vi "EntêteFichierTlog.vi"(3 "Error in":errorcluster, 4 "TSensPAr":T1[](array[typedef]) {"Compensation" items=["Off", "On"]; "TableConv" max=60 step=1; "Type" items=["Silicon Diode", "GaAlAs Diode", "Platinum 100 (250 Ohms)", "Platinum 100 (500 Ohms)", "Platinum 1000 Ohms", "NTC RTD 75mV 7.5 KOhms", "Thermocouple 25mV", "Thermocouple 50mV", "NTC RTD 75mV 75 Ohms", "NTC RTD 75mV 750 Ohms", "NTC RTD 75mV 7.5 KOhms", "NTC RTD 75mV 75 KOhms", "NTC RTD 75mV Auto"]; "TableTC" max=41 step=1}, 5 "ConfigChoisies":string[](array[string]) caption="Configurations\nChoisies") -> (0 "error out":errorcluster, 1 "Entête":string, 2 "Scan list Out":string[](array[string]))   [LabVIEW 2010]
doc: "Ce Vi créer la ligne d'entête du fichier texte de sauvegarde à partir du nombre de paramètre voulus."
uses:
  <userlib>/LSCI 332/LSCI332.llb/InConfigPar332.ctl
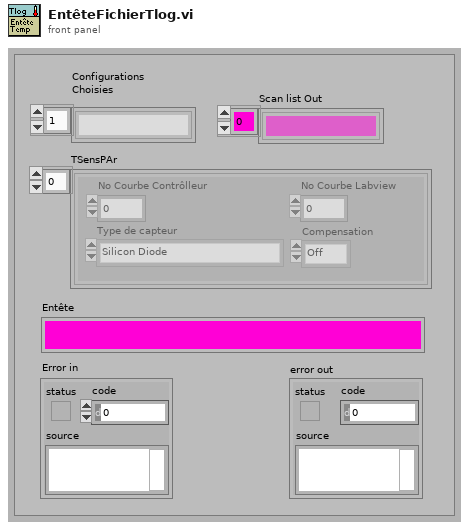
[diagram p1: front panel]
types:
  T1 = typedef "InConfigPar332.ctl" = cluster{"TableTC":u16, "TableConv":u16, "Compensation":u16, "Type":u16}
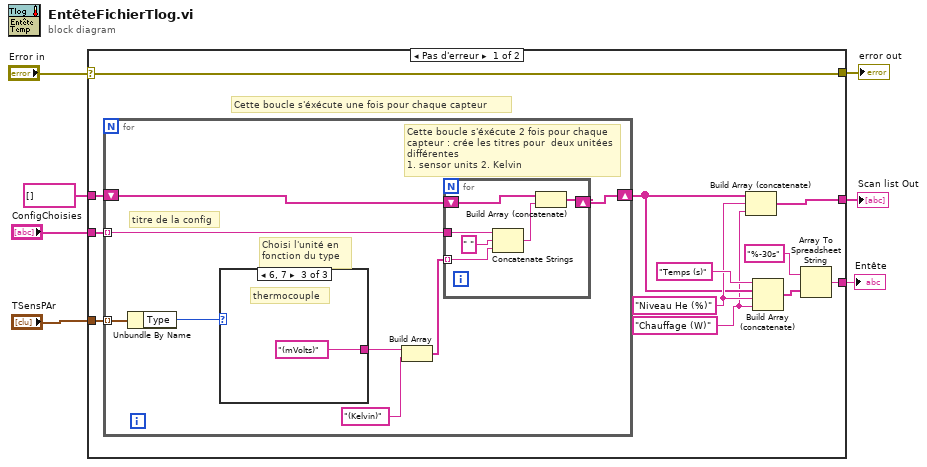
[diagram p0: block diagram]
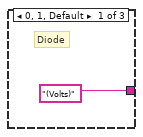
[diagram p2: hidden frame]
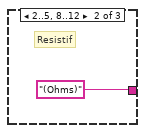
[diagram p3: hidden frame]
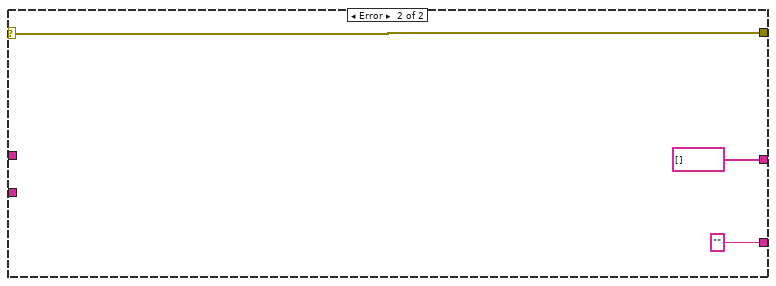
[diagram p4: hidden frame]
diagram:
  n1 = case shown="Pas d'erreur" "Error in" {
    selector: "Error in" -> [w9 w38]
    tunnel: "ConfigChoisies" -> [w19 _]
    tunnel: [w15 "" ("spreadsheet string")] -> w6
    tunnel: [w9 w38] -> w4
    tunnel: [w12 string[] []] -> w3
    tunnel: "TSensPAr" -> [w11 _]
    tunnel: string[] [] -> [w10 _]
    frame No Error {
      w8 = "Chauffage (W)"
      w14 = "Niveau He (%)"
      # "Cette boucle s'éxécute une fois pour chaque capteur"
      n2 = for {
        tunnel: w19 -> [w25] mode=indexing
        shift-right: [w27] -> w13
        shift-left: w10 -> [w26]
        tunnel: w11 -> [w24] mode=indexing
        # "Cette boucle s'éxécute 2 fois pour chaque capteur : crée les titres pour  deux unitées différentes \n1. sensor units 2. Kelvin"
        # "Choisi l'unité en\nfonction du type"
        # "titre de la config"
        n3 = Unbundle By Name(w24) -> ("Type"=w20:u16)
        n4 = case shown="6, 7" w20 {
          tunnel: ["(Volts)" "(Ohms)" "(mVolts)"] -> w23
          frame 0, 1, Default {
            # "Diode"
          }
          frame 2..5, 8..12 {
            # "Resistif"
          }
          frame 6, 7 {
            # "thermocouple"
          }
        }
        n5 = Build Array(w23, "(Kelvin)") -> (w21:string[])
        n6 = for {
          tunnel: w25 -> [w36]
          shift-right: [w35] -> w27
          shift-left: w26 -> [w34]
          tunnel: w21 -> [w31] mode=indexing
          n7 = Concatenate Strings(w36, " ", w31) -> (w32:string)
          n8 = Build Array (concatenate)(w34, w32) -> (w35:string[])
        }
      }
      n9 = Build Array (concatenate)(w13, w14, w8) -> (w12:string[])
      n10 = Build Array (concatenate)("Temps (s)", w13, w14, w8) -> (w17:string[])
      n11 = Array To Spreadsheet String(array=w17, 3:"%-30s" ("format string")) -> (spreadsheet string=w15:string)  [unwired: 1 in]
    }
    frame Error {
    }
  }
  "Scan list Out" <- w3
  "Entête" <- w6
  "error out" <- w4
